vi "do domu sprobowac.vi"() -> ()   [LabVIEW 2023]
panel:
  in  "pokazanie liczby":T1(ring)
  out "Numeric":dbl
  in  "c":dbl
  in  "b":dbl
  in  "a":dbl
  in  "x":dbl
  in  "y = a +bx + cx^2":bool
  # "y = a + bx^2 - 3x^4"
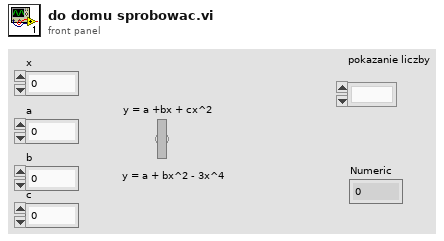
[diagram p1: front panel]
types:
  T1 = enum16{"", "dziesietny", "osemkowy", "szestnastkowy\n"}
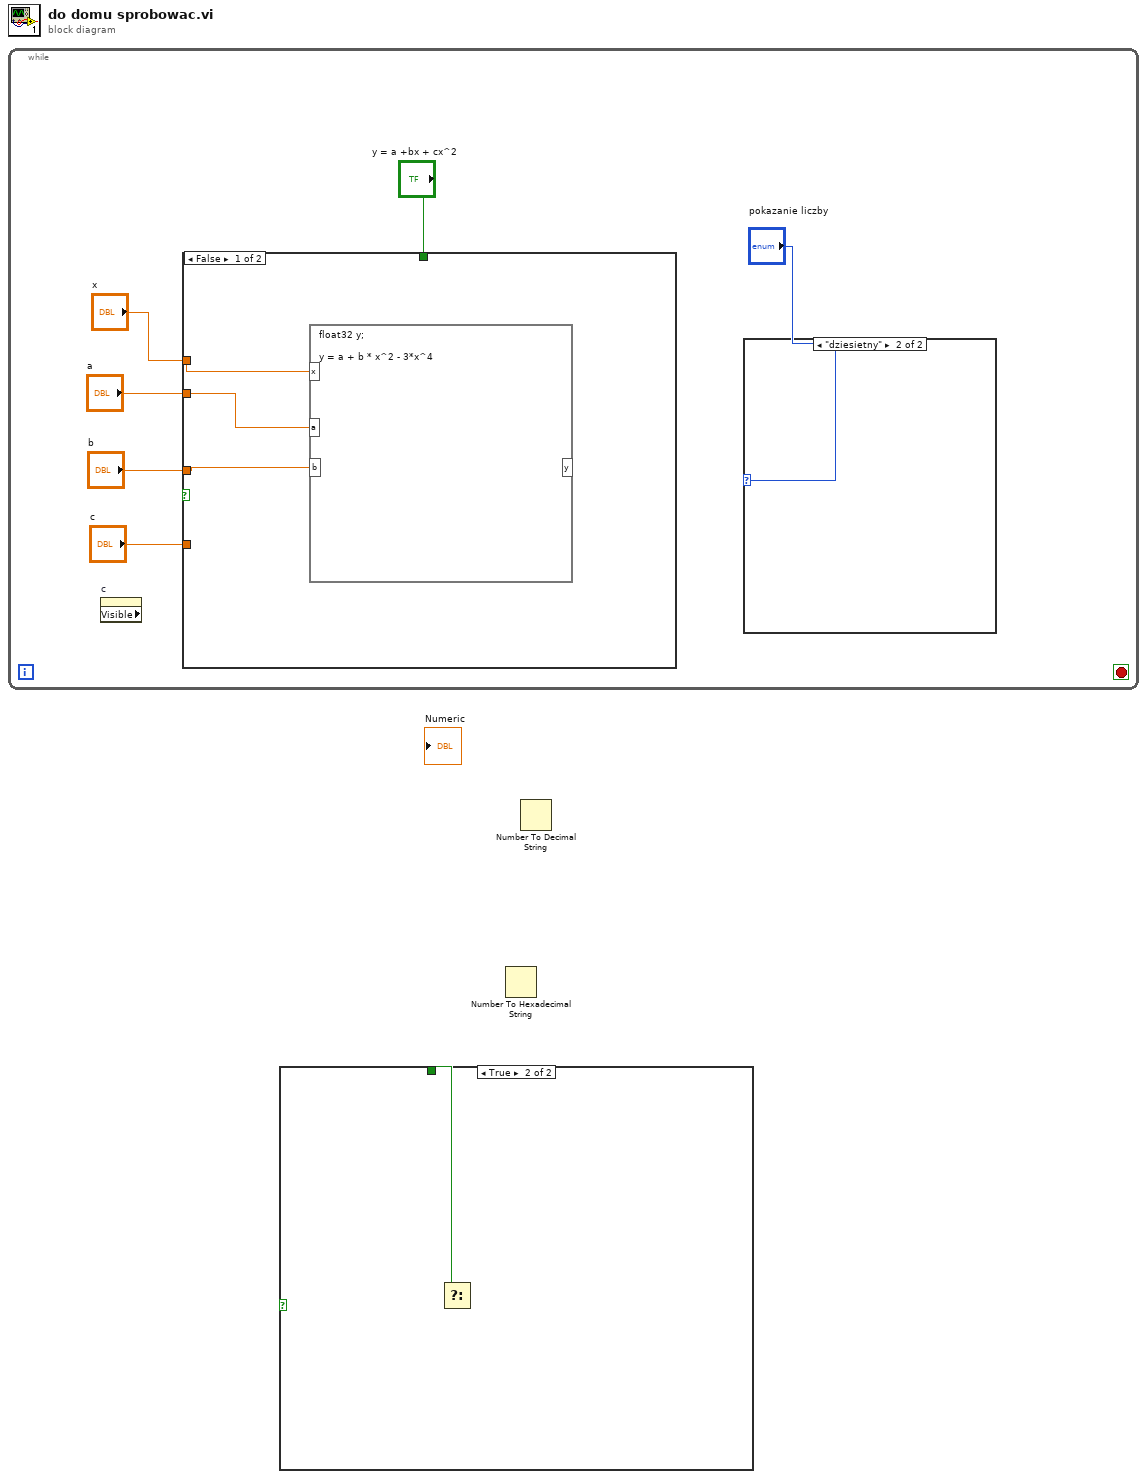
[diagram p0: block diagram]
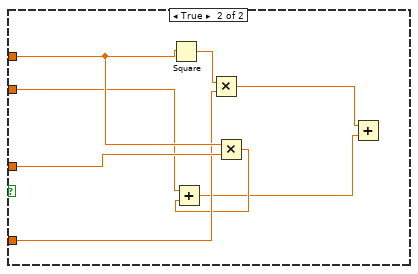
[diagram p3: hidden frame]
diagram:
  n1 = while {
    stop <- _ stop-if-true
    n2 = property on="c" class="DigNum (strict)" props=["Visible"]() -> ()  [unwired: 2 in, 3 out]
    n3 = case shown="False" {
      selector: _ -> [_ _]
      tunnel: "b" -> [w8 w18]
      tunnel: "x" -> [w10 w17]
      tunnel: "c" -> [_ w16]
      tunnel: "a" -> [w9 w14]
      tunnel: "y = a +bx + cx^2" -> [_ _]
      frame False {
        n4 = formula code="float32 y;\n\ny = a + b * x^2 - 3*x^4"("x"=w10, "a"=w9, "b"=w8) -> ()  [unwired: 1 out]
      }
      frame True {
        n5 = Square(x=w17) -> (x^2=w15:dbl)
        n6 = Multiply(x=w15, y=w16) -> (x*y=w11:dbl)
        n7 = Multiply(x=w17, y=w18) -> (x*y=w13:dbl)
        n8 = Add(x=w14, y=w13) -> (x+y=w12:dbl)
        n9 = Add(x=w11, y=w12) -> ()  [unwired: 1 out]
      }
    }
    n10 = case shown="\"dziesietny\"" "pokazanie liczby" {
      frame "", Default {
      }
      frame "dziesietny" {
      }
    }
  }
  n11 = case shown="True" {
    selector: _ -> [_ _]
    tunnel: [_ w19] -> w1
    frame False {
    }
    frame True {
      n12 = Select(s=w19) -> ()  [unwired: 2 in, 1 out]
    }
  }
  n13 = Number To Hexadecimal String() -> ()  [unwired: 2 in, 1 out]
  n14 = Number To Decimal String() -> ()  [unwired: 2 in, 1 out]
